vi "correctAllDelays.vi"(8 "error in (no error)":errorcluster, 11 "ScriptEventList in":refnum<class "ScriptEventList.lvclass">) -> (0 "error out":errorcluster, 3 "ScriptEventList out":refnum<class "ScriptEventList.lvclass">)   [LabVIEW 2009, in "Tools.lvlib" / "Scripting.lvlib" / "ScriptEventList.lvclass"]
uses:
  ScriptEventList.lvclass
  ScriptEventList.lvclass/ScriptEventList.ctl
  ScriptEvent.lvclass
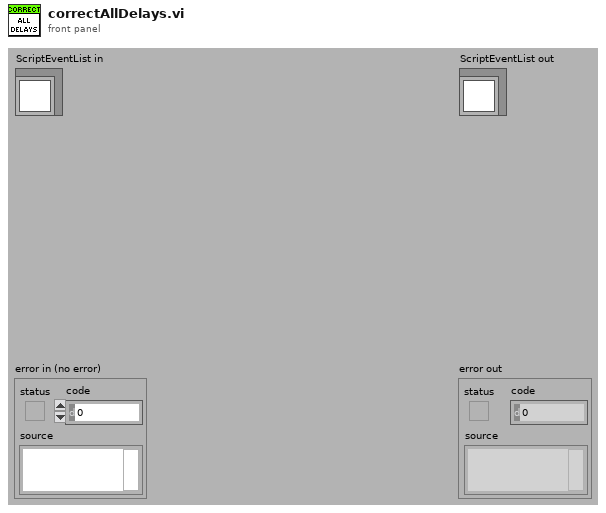
[diagram p1: front panel]
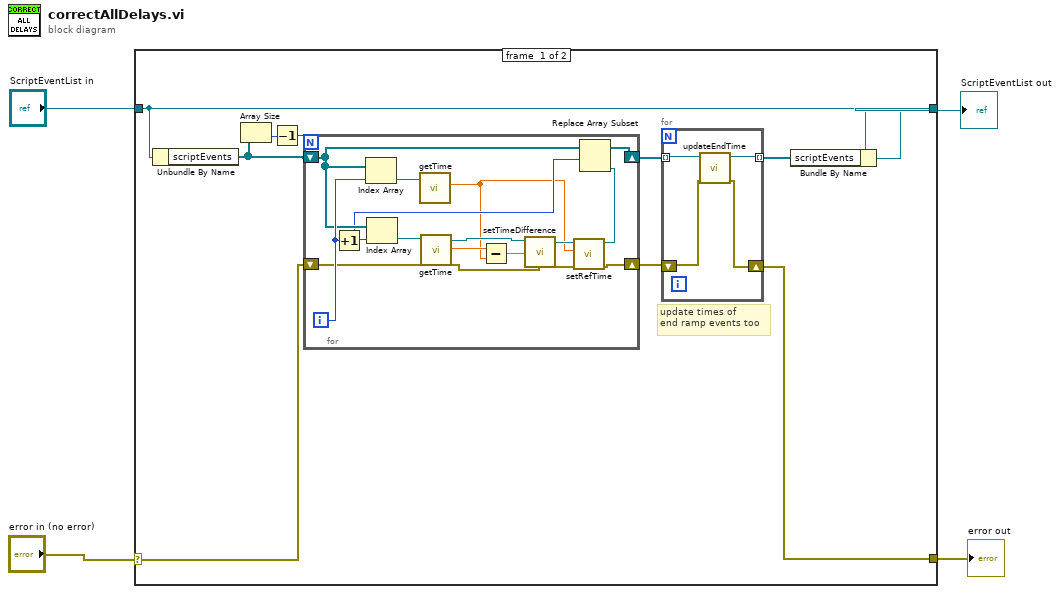
[diagram p0: block diagram]
diagram:
  n1 = case shown="No Error" "error in (no error)" {
    selector: "error in (no error)" -> [w9 w36]
    tunnel: [w5 w36] -> w3
    tunnel: [w10 w35] -> w1
    tunnel: "ScriptEventList in" -> [w11 w35]
    frame #0 {
      # "update times of\nend ramp events too"
      n2 = Unbundle By Name(w11) -> ("scriptEvents"=w14:refnum<class "ScriptEvent.lvclass">[])
      n3 = Array Size(array=w14) -> (size(s)=w13:i32)
      n4 = Decrement(x=w13) -> (x-1=w12:i32)
      n5 = for {
        N: w12 -> [_]
        shift-right: [w24] -> w7
        shift-left: w14 -> [w28]
        shift-right: [w23] -> w6
        shift-left: w9 -> [w27]
        i -> [w34]
        n6 = Increment(x=w34) -> (x+1=w25:i32)
        n7 = Index Array(array=w28, index=w34) -> (element=w33:refnum<class "ScriptEvent.lvclass">)
        n8 = Index Array(array=w28, index=w25) -> (element=w32:refnum<class "ScriptEvent.lvclass">)
        n9 = call "getTime.vi"("ScriptEvent.lvclass in"=w33) -> ("time"=w20:dbl)  [unwired: 8 in, 2 out]
        n10 = call "getTime.vi"("error in (no error)"=w27, "ScriptEvent.lvclass in"=w32) -> ("error out"=w29:errorcluster, "time"=w31:dbl, "ScriptEvent.lvclass out"=w30:refnum<class "ScriptEvent.lvclass">)  [unwired: 7 in]
        n11 = Subtract(x=w31, y=w20) -> (x-y=w26:dbl)
        n12 = call "setTimeDifference.vi"("error in (no error)"=w29, "time difference"=w26, "ScriptEvent.lvclass in"=w30) -> ("error out"=w22:errorcluster, "ScriptEvent.lvclass out"=w21:refnum<class "ScriptEvent.lvclass">)  [unwired: 7 in]
        n13 = call "setRefTime.vi"("error in (no error)"=w22, "refTime"=w20, "ScriptEvent.lvclass in"=w21) -> ("error out"=w23:errorcluster, "ScriptEvent.lvclass out"=w19:refnum<class "ScriptEvent.lvclass">)  [unwired: 7 in]
        n14 = Replace Array Subset(array=w28, new element=w19, index=w25) -> (w24:refnum<class "ScriptEvent.lvclass">[])
      }
      n15 = for {
        tunnel: [w18] -> w8 mode=indexing
        tunnel: w7 -> [w17] mode=indexing
        shift-right: [w15] -> w5
        shift-left: w6 -> [w16]
        n16 = call-dynamic "updateEndTime.vi"("error in (no error)"=w16, "ScriptEvent in"=w17) -> ("error out"=w15:errorcluster, "ScriptEvent out"=w18:refnum<class "ScriptEvent.lvclass">)  [unwired: 8 in]
      }
      n17 = Bundle By Name(cluster=w11, "scriptEvents"=w8) -> (w10:refnum<class "ScriptEventList.lvclass">)
    }
    frame #1 {
    }
  }
  "error out" <- w3
  "ScriptEventList out" <- w1
